vi "DB List Tables.vi"(8 "error in (no error)":errorcluster, 11 "MYSQL Database in":refnum<class "MYSQL Server.lvclass">) -> (0 "error out":errorcluster, 2 "tables":string[](array[string]), 3 "MYSQL Database out":refnum<class "MYSQL Server.lvclass">)   [LabVIEW 2023, in "HardwareAbstractionLayer_LVOOP.lvlib" / "MYSQL Server.lvclass"]
uses:
  MYSQL Server.lvclass
  MYSQL Server.lvclass/MYSQL Server.ctl
  <vilib>/addons/database/NI_Database_API.lvlib
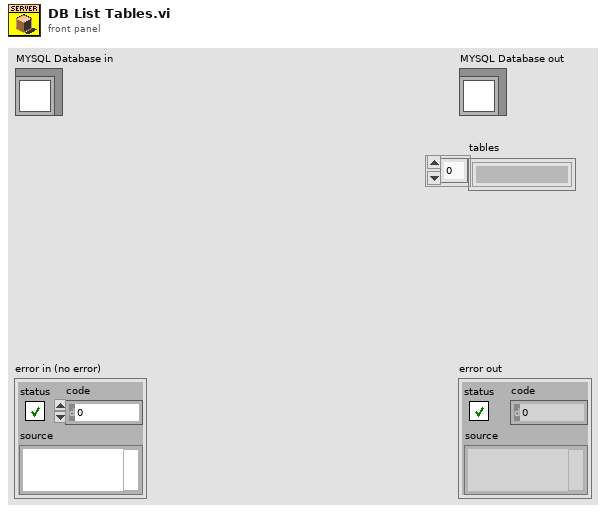
[diagram p1: front panel]
types:
  T1 = typedef "NI_Database_API.lvlib/Conn ObjectReference.ctl" = refnum<k1>
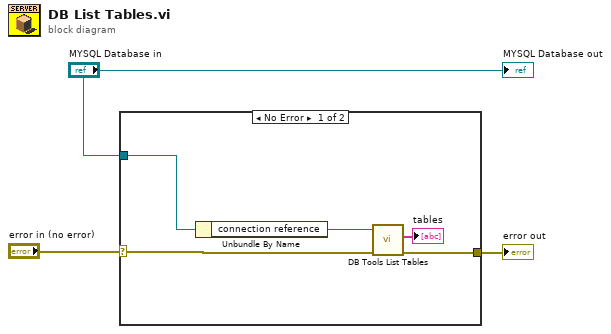
[diagram p0: block diagram]
diagram:
  n1 = case shown="No Error" "error in (no error)" {
    selector: "error in (no error)" -> [w6 w9]
    tunnel: "MYSQL Database in" -> [w8 _]
    tunnel: [w5 w9] -> w1
    frame No Error {
      n2 = Unbundle By Name(w8) -> ("connection reference"=w7:T1)
      n3 = call <vilib>:"DB Tools List Tables.vi"("error in (no error)"=w6, "connection reference"=w7) -> ("error out"=w5:errorcluster, "tables"=→"tables":string[])  [unwired: 3 in, 1 out]
    }
    frame Error {
    }
  }
  "error out" <- w1
  "MYSQL Database out" <- "MYSQL Database in"
